vi "Configure Data Acquisition.vi"(7 "Enable Trigged Acquistion (False)":bool, 8 "error in (no error)":errorcluster, 9 "Sample Rate (0.001)":dbl=0.001 min=0.0002 max=800000.0, 10 "Enable Acquisition State (False)":bool, 11 "VISA resource name":refnum<visa-resource-name>) -> (0 "error out":errorcluster, 3 "VISA resource name out":refnum<visa-resource-name>)   [LabVIEW 2017, in "HH PLI Series.lvlib"]
doc: "Configures data acquisition in static operation mode.\n\n<b>Note</b>\nThe measurement data is saved in the internal instrument memory.\nThe internal instrument memory can save up to 8000 measurement data points."
uses:
  HH PLI Series.lvlib
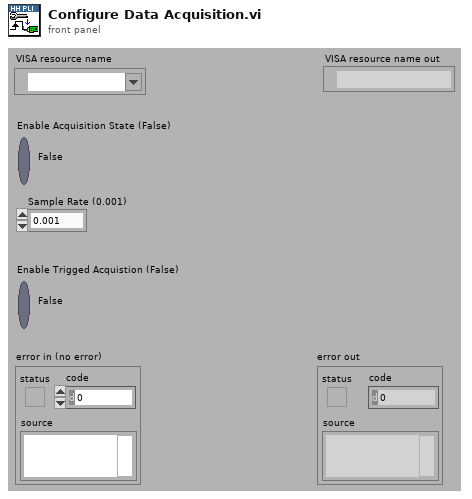
[diagram p1: front panel]
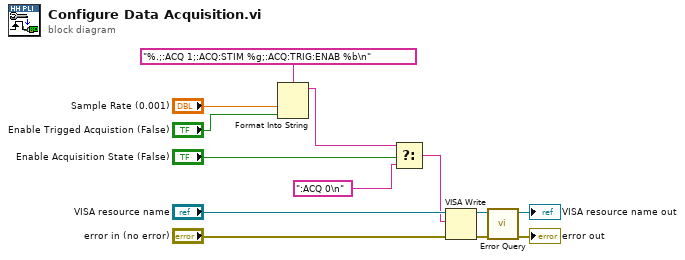
[diagram p0: block diagram]
diagram:
  n1 = Format Into String(format string="%.;:ACQ 1;:ACQ:STIM %g;:ACQ:TRIG:ENAB %b\n", "Sample Rate (0.001)", "Enable Trigged Acquistion (False)") -> (resulting string=w4:string)  [unwired: 2 in, 1 out]
  n2 = Select(t=w4, s="Enable Acquisition State (False)", f=":ACQ 0\n") -> (s? t:f=w1:string)
  n3 = VISA Write(VISA resource name="VISA resource name", write buffer=w1, error in (no error)="error in (no error)") -> (VISA resource name out=w11:refnum<visa-resource-name>, error out=w12:errorcluster)  [unwired: 1 out]
  n4 = call "Error Query.vi"("error in (no error)"=w12, "VISA resource name"=w11) -> ("error out"=→"error out":errorcluster, "VISA resource name out"=→"VISA resource name out":refnum<visa-resource-name>)  [unwired: 6 in, 2 out]
